vi "最大值比较器（DBL).vi"(10 "reset":bool, 11 "Input":dbl) -> (3 "Max":dbl)   [LabVIEW 2012]
doc: "功能：\n\n根据输入的数值，连续比较输入的最大值。\n\n基本算法：\n\n利用LV2全局变量（反馈节点）存储上一次输入值，和本次输入值比较，返回最大值。\n\nCSXCS_366创建"
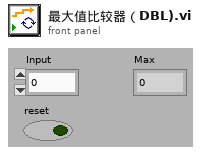
[diagram p1: front panel]
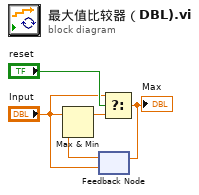
[diagram p0: block diagram]
diagram:
  n1 = feedback #1("Input") -> (w5:dbl)
  n2 = Max & Min(x="Input", y=w5) -> (max(x,y)=w3:dbl)  [unwired: 1 out]
  n3 = Select(t="Input", s="reset", f=w3) -> (s? t:f=w4:dbl)
  "Max" <- w4
  n4 = feedback-in #1(w4) -> ()
